vi "ASI Get ROI Format.vi"(6 "pImg_type":i32, 7 "piBin":i32, 9 "piHeight":i32, 10 "piWidth":i32, 11 "iCameraID":i32) -> (1 "piHeight out":i32, 2 "piWidth out":i32, 3 "function return":i32, 4 "pImg_type out":i32, 5 "piBin out":i32)   [LabVIEW 2012, in "ASICamera2_no_err.lvlib"]
doc: "ASICAMERA_API ASI_ERROR_CODE ASIGetROIFormat(int iCameraID, int *piWidth, int *piHeight, int *piBin, ASI_IMG_TYPE *pImg_type);"
uses:
  <userlib>/ASICamera2_no_err/ASICamera2_no_err.lvlib
  ASICamera2.dll
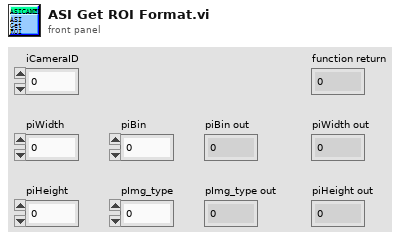
[diagram p1: front panel]
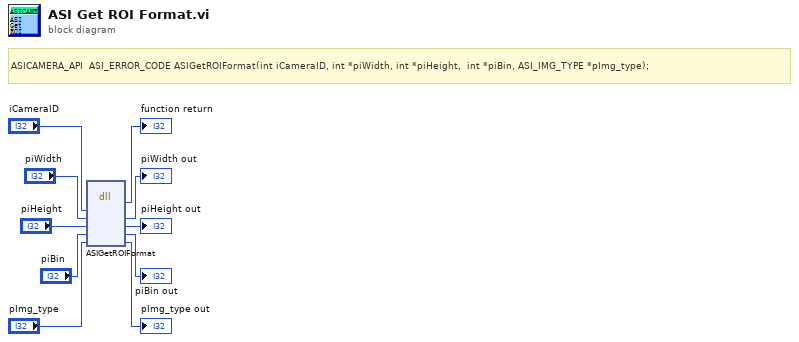
[diagram p0: block diagram]
diagram:
  # "ASICAMERA_API  ASI_ERROR_CODE ASIGetROIFormat(int iCameraID, int *piWidth, int *piHeight,  int *piBin, ASI_IMG_TYPE *pImg_type);"
  n1 = dll-call lib="ASICamera2.*" fn="ASIGetROIFormat"("iCameraID"="iCameraID", "piWidth"="piWidth", "piHeight"="piHeight", "piBin"="piBin", "pImg_type"="pImg_type") -> (→"function return":i32, "piWidth"=→"piWidth out":i32, "piHeight"=→"piHeight out":i32, "piBin"=→"piBin out":i32, "pImg_type"=→"pImg_type out":i32)  [unwired: 4 in, 2 out]
